vi "Test API if the vi pane control refs are cluster and they are parsed correctly.vi"(8 "error in":errorcluster, 11 "TestCase in":refnum<class "Test Scripting API.lvclass">) -> (0 "error out":errorcluster, 3 "TestCase out":refnum<class "Test Scripting API.lvclass">)   [LabVIEW 2020, in "Test Scripting API.lvclass"]
uses:
  Test Scripting API.lvclass
  <vilib>/Utility/Data Type/Type Definitions/Data Type.ctl
  VI UUT_Complex.vi
  Scripting Playground/Scripting/DQMH_API.lvlib
  <vilib>/Utility/Data Type/NI_Data Type.lvlib
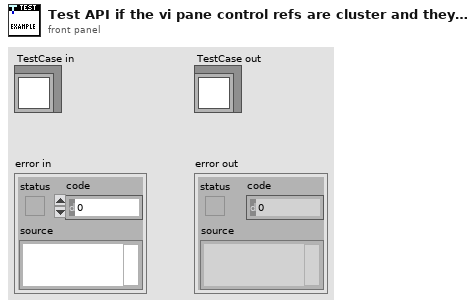
[diagram p1: front panel]
types:
  T1 = typedef "NI_Data Type.lvlib/Data Type.ctl" = enum8{"Invalid Type", "Void", "I8", "I16", "I32", "I64", "U8", "U16", "U32", "U64", "Single Float", "Double Float", "Extended Float", "Single Complex", "Double Complex", "Extended Complex", "Enum U8", "Enum U16", "Enum U32", "Enum U64", "Single Float With Unit", "Double Float With Unit", "Extended Float With Unit", "Single Complex with Unit", "Double Complex with Unit", "Extended Complex with Unit", "Boolean", "String", "Path", "Picture", "Tag", "Array", "Cluster", "Variant", "LV Variant", "Waveform", "Timestamp", "Digital Waveform", "Digital Data", "ExpressData", "Refnum", "External Data", "VI", "Poly VI", "LabVIEW Class Instance", "Fixed Point", "Set Collection", "Map Collection"}
  T2 = typedef "DQMH_API.lvlib/Controls Refs and Type--cluster.ctl" = cluster{"Ctrls Refs ":refnum<vi>[], "Ctrls Types":T1[], "Names":string[]}
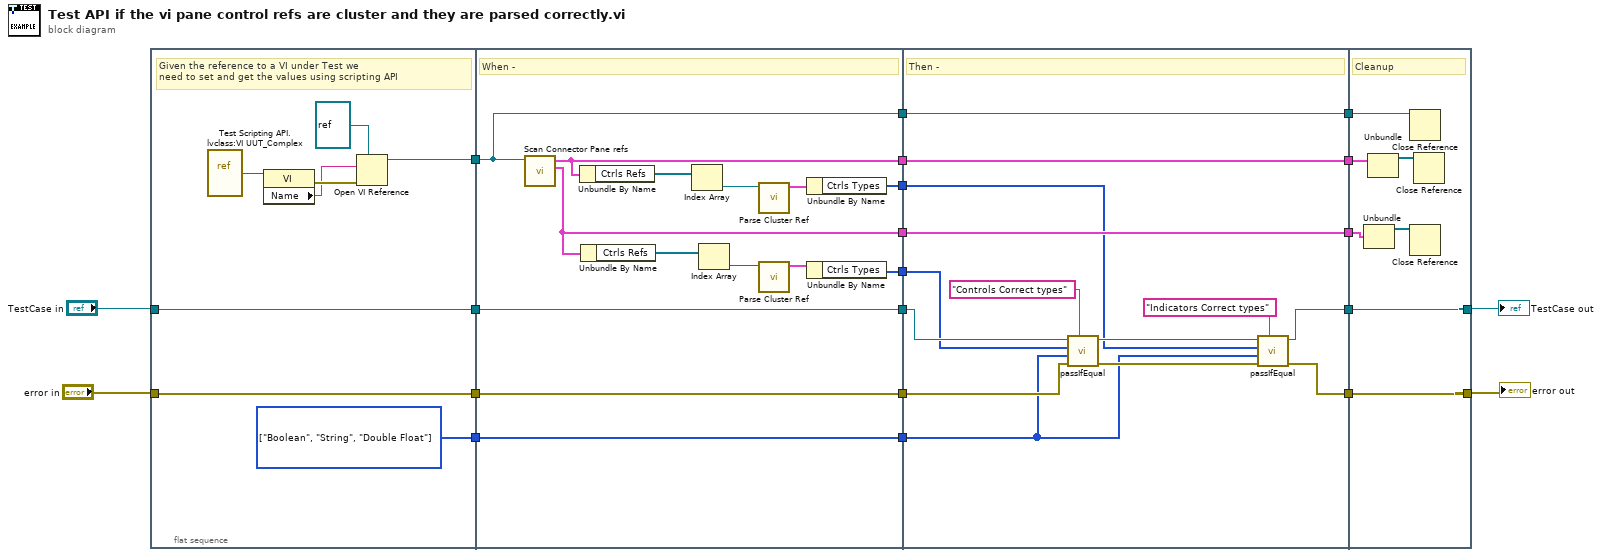
[diagram p0: block diagram]
diagram:
  n1 = flat-sequence {
    tunnel: "error in" -> [w29]
    tunnel: "TestCase in" -> [w27]
    tunnel: [w27] -> w16
    tunnel: [w29] -> w21
    tunnel: [w23] -> w10
    tunnel: [w22] -> w3
    tunnel: [w42] -> w15
    tunnel: [w43] -> w20
    tunnel: w16 -> [w42]
    tunnel: w21 -> [w43]
    tunnel: [w39] -> w11
    tunnel: w10 -> [w41]
    tunnel: [w41] -> w9
    tunnel: [w40] -> w5
    tunnel: [w38] -> w4
    tunnel: w3 -> [w38]
    tunnel: [w31] -> w2
    tunnel: [w30] -> w1
    tunnel: [w52] -> w14
    tunnel: [w55] -> w19
    tunnel: w15 -> [w54]
    tunnel: w20 -> [w57]
    tunnel: w11 -> [w50]
    tunnel: w9 -> [w51]
    tunnel: [w51] -> w8
    tunnel: [w50] -> w7
    tunnel: [w49] -> w6
    tunnel: w5 -> [w49]
    tunnel: w4 -> [w48]
    tunnel: w2 -> [w45]
    tunnel: w1 -> [w44]
    tunnel: [w64] -> w17
    tunnel: [w63] -> w12
    tunnel: w14 -> [w63]
    tunnel: w19 -> [w64]
    tunnel: w8 -> [w62]
    tunnel: w7 -> [w60]
    tunnel: w6 -> [w61]
    frame #0 {
      w22 = T1[] [enum."Boolean", enum."String", enum."Double Float"] items=["Invalid Type", "Void", "I8", "I16", "I32", "I64", "U8", "U16", "U32", "U64", "Single Float", "Double Float", "Extended Float", "Single Complex", "Double Complex", "Extended Complex", "Enum U8", "Enum U16", "Enum U32", "Enum U64", "Single Float With Unit", "Double Float With Unit", "Extended Float With Unit", "Single Complex with Unit", "Double Complex with Unit", "Extended Complex with Unit", "Boolean", "String", "Path", "Picture", "Tag", "Array", "Cluster", "Variant", "LV Variant", "Waveform", "Timestamp", "Digital Waveform", "Digital Data", "ExpressData", "Refnum", "External Data", "VI", "Poly VI", "LabVIEW Class Instance", "Fixed Point", "Set Collection", "Map Collection"] ("Ctrls Types")
      # "Given the reference to a VI under Test we\nneed to set and get the values using scripting API"
      n2 = vi-ref "Test Scripting API.lvclass:VI UUT_Complex.vi"() -> (w26:refnum<vi>)
      n3 = property class="VI"(reference=w26) -> (error out=w28:errorcluster, "Name"=w25:string)  [unwired: 1 in, 1 out]
      n4 = Open VI Reference(type specifier VI Refnum (for type only)=refnum<vi> refnum, vi path=w25, error in (no error)=w28) -> (vi reference=w23:refnum<vi>)  [unwired: 3 in, 1 out]
    }
    frame #1 {
      # "When -"
      n5 = call "Scan Connector Pane refs.vi"("VI in"=w41) -> ("Controls"=w40:T2, "Indicators"=w39:T2)  [unwired: 9 in]
      n6 = Unbundle By Name(w39) -> ("Ctrls Refs"=w37:refnum<vi>[])
      n7 = Unbundle By Name(w40) -> ("Ctrls Refs"=w36:refnum<vi>[])
      n8 = Index Array(array=w37) -> (element=w35:refnum<vi>)  [unwired: 1 in]
      n9 = Index Array(array=w36) -> (element=w34:refnum<vi>)  [unwired: 1 in]
      n10 = call "Parse Cluster Ref.vi"("Cluster Ref"=w35) -> ("Controls Refs and Types"=w33:T2)  [unwired: 10 in]
      n11 = call "Parse Cluster Ref.vi"("Cluster Ref"=w34) -> ("Controls Refs and Types"=w32:T2)  [unwired: 10 in]
      n12 = Unbundle By Name(w33) -> ("Ctrls Types"=w31:T1[])
      n13 = Unbundle By Name(w32) -> ("Ctrls Types"=w30:T1[])
    }
    frame #2 {
      # "Then -"
      n14 = call-dynamic "passIfEqual.vi"("custom report message (\"\")"="Controls Correct types" ("custom report message (\"\")"), "error in (no error)"=w57, "y"=w48, "x"=w44, "TestCase in"=w54) -> ("error out"=w56:errorcluster, "TestCase out"=w53:refnum<class "Test Scripting API.lvclass">)  [unwired: 5 in]
      n15 = call-dynamic "passIfEqual.vi"("custom report message (\"\")"="Indicators Correct types" ("custom report message (\"\")"), "error in (no error)"=w56, "y"=w48, "x"=w45, "TestCase in"=w53) -> ("error out"=w55:errorcluster, "TestCase out"=w52:refnum<class "Test Scripting API.lvclass">)  [unwired: 5 in]
    }
    frame #3 {
      # "Cleanup"
      n16 = Unbundle(w61) -> ("Ctrls Refs"=w58:refnum<vi>[])  [unwired: 2 out]
      n17 = Unbundle(w60) -> ("Ctrls Refs"=w59:refnum<vi>[])  [unwired: 2 out]
      n18 = Close Reference(reference=w62) -> ()  [unwired: 1 in, 1 out]
      n19 = Close Reference(reference=w58) -> ()  [unwired: 1 in, 1 out]
      n20 = Close Reference(reference=w59) -> ()  [unwired: 1 in, 1 out]
    }
  }
  "error out" <- w17
  "TestCase out" <- w12
